vi "Updater Spartan INI.vi"(8 "error in (no error)":errorcluster, 10 "Spartan Server.ini":path, 11 "Copy Keys From INI":path) -> (0 "error out":errorcluster, 3 "Run as Service?":bool)   [LabVIEW 2011]
uses:
  Summitek EXT/OpenG EXT/file/file.llb/Valid Path - Traditional__ogtk.vi
  Summitek EXT/OpenG EXT/file/file.llb/File Exists - Scalar__ogtk.vi
  <vilib>/Utility/config.llb/Read Key (Boolean).vi
  <vilib>/Utility/config.llb/Read Key (String).vi
  <vilib>/Utility/config.llb/Write Key (String).vi
  <vilib>/Utility/config.llb/NI_LVConfig.lvlib
panel:
  # "This VI should run from TARGET root (e.g., \"<Program Files>\\Summitek\\Spartan\\\")\nwhenever the updater.exe runs.  It is used to put the \"Default Configuration.ini\"\ninto the \"Spartan Server.ini\" (while maintaining any previous relevant config values)."
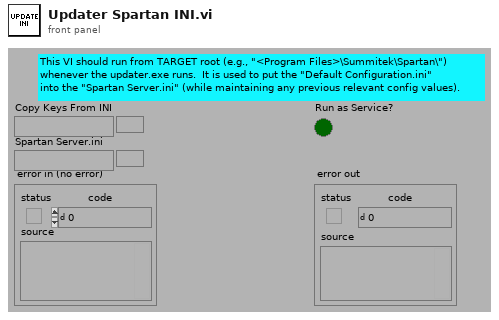
[diagram p1: front panel]
types:
  T1 = cluster{"Section":string, "Key":string, "Value":string}[]
  T2 = typedef "NI_LVConfig.lvlib/Config Data RefNum.ctl" = refnum<k1>
  T3 = cluster{"String":string, "String":string, "value":string}
  T4 = cluster{"String":string, "String":string, "value":string}[]
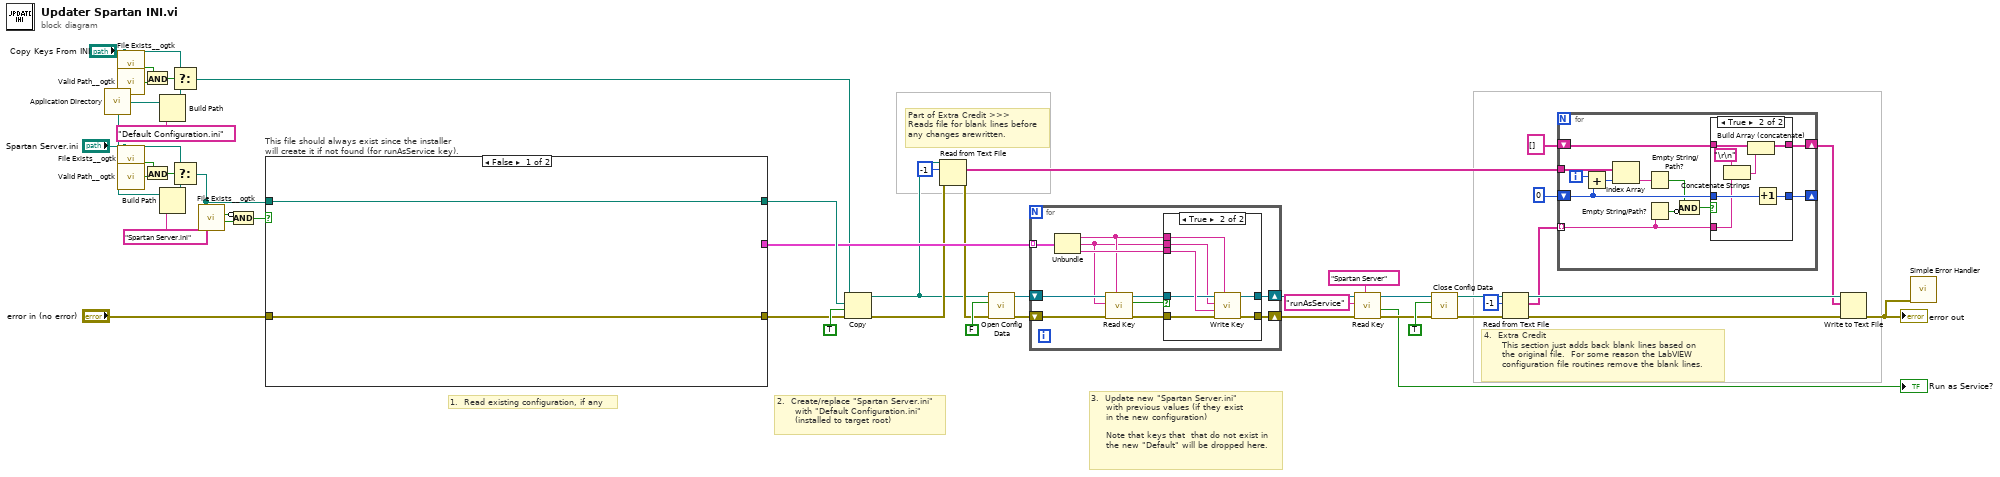
[diagram p0: block diagram]
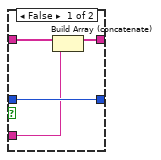
[diagram p2: hidden frame]
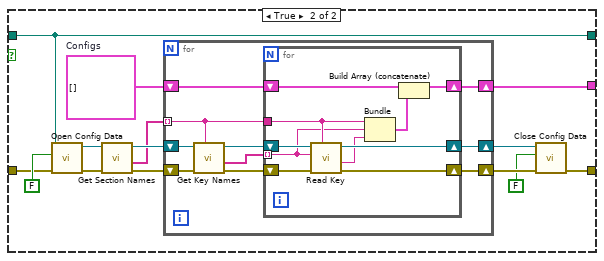
[diagram p4: hidden frame]
diagram:
  # "Part of Extra Credit >>>\nReads file for blank lines before\nany changes arewritten."
  # "4.  Extra Credit\n      This section just adds back blank lines based on\n      the original file.  For some reason the LabVIEW\n      configuration file routines remove the blank lines."
  # "3.  Update new \"Spartan Server.ini\"\n     with previous values (if they exist\n     in the new configuration)\n\n     Note that keys that  that do not exist in\n     the new \"Default\" will be dropped here."
  # "2.  Create/replace \"Spartan Server.ini\"\n      with \"Default Configuration.ini\"\n      (installed to target root)"
  # "1.  Read existing configuration, if any"
  n1 = call <vilib>:"Application Directory.vi"() -> ("Application Directory"=w14:path)
  n2 = call-poly "File Exists__ogtk.vi"("file path"="Copy Keys From INI") -> ("exists"=w7:bool)  [unwired: 6 in, 1 out]
  n3 = call-poly "Valid Path__ogtk.vi"("path"="Copy Keys From INI") -> ("valid"=w8:bool)
  n4 = call-poly "File Exists__ogtk.vi"("file path"="Spartan Server.ini") -> ("exists"=w5:bool)  [unwired: 6 in, 1 out]
  n5 = call-poly "Valid Path__ogtk.vi"("path"="Spartan Server.ini") -> ("valid"=w4:bool)
  n6 = And(x=w7, y=w8) -> (x .and. y?=w6:bool)
  n7 = And(x=w5, y=w4) -> (x .and. y?=w3:bool)
  n8 = Build Path(base path=w14, name or relative path="Default Configuration.ini") -> (appended path=w13:path)
  n9 = Build Path(base path=w14, name or relative path="Spartan Server.ini") -> (appended path=w11:path)
  n10 = Select(t="Copy Keys From INI", s=w6, f=w13) -> (s? t:f=w12:path)
  n11 = Select(t="Spartan Server.ini", s=w3, f=w11) -> (s? t:f=w10:path)
  n12 = call-poly "File Exists__ogtk.vi"("file path"=w10) -> ("is directory"=w47:bool, "exists"=w46:bool)  [unwired: 6 in]
  n13 = Compound Arithmetic op=AND(invert w47, w46) -> (w44:bool)
  n14 = case "This file should always exist since the installer will create it if not found (for runAsService key)." shown="False" w44 {
    tunnel: w10 -> [w49 w51]
    tunnel: "error in (no error)" -> [w50 w63]
    tunnel: [w50 w56] -> w41
    tunnel: [_ w52] -> w37
    tunnel: [w49 w51] -> w40
    frame False {
    }
    frame True {
      w53 = T1 []  # Configs
      n15 = call <vilib>:"Open Config Data.vi"("error in (no error)"=w63, "create file if necessary (T)"=FALSE, "configuration file path"=w51) -> ("error out"=w61:errorcluster, "refnum"=w62:T2)  [unwired: 6 in, 1 out]
      n16 = call <vilib>:"Get Section Names.vi"("error in (no error)"=w61, "refnum"=w62) -> ("error out"=w60:errorcluster, "section names"=w58:string[], "refnum out"=w59:T2)  [unwired: 7 in]
      n17 = for {
        shift-right: [w69] -> w57
        shift-left: w60 -> [w73]
        shift-right: [w70] -> w55
        shift-left: w59 -> [w74]
        tunnel: w58 -> [w68] mode=indexing
        shift-right: [w65] -> w52
        shift-left: w53 -> [w66]
        n18 = call <vilib>:"Get Key Names.vi"("section"=w68, "error in (no error)"=w73, "refnum"=w74) -> ("error out"=w71:errorcluster, "key names"=w67:string[], "refnum out"=w72:T2)  [unwired: 5 in, 1 out]
        n19 = for {
          shift-right: [w82] -> w69
          shift-left: w71 -> [w83]
          shift-right: [w81] -> w70
          shift-left: w72 -> [w84]
          tunnel: w68 -> [w80]
          tunnel: w67 -> [w79] mode=indexing
          shift-right: [w76] -> w65
          shift-left: w66 -> [w77]
          n20 = call-poly <vilib>:"Read Key.vi"("section"=w80, "error in (no error)"=w83, "key"=w79, "refnum"=w84) -> ("error out"=w82:errorcluster, "value"=w78:string, "refnum out"=w81:T2)  [unwired: 4 in, 1 out]
          n21 = Bundle("String"=w80, "String"=w79, "value"=w78) -> (w75:T3)  [unwired: 1 in]
          n22 = Build Array (concatenate)(w77, w75) -> (w76:T4)
        }
      }
      n23 = call <vilib>:"Close Config Data.vi"("error in (no error)"=w57, "write file if changed (T)"=FALSE, "refnum"=w55) -> ("error out"=w56:errorcluster)  [unwired: 7 in, 1 out]
    }
  }
  n24 = Copy(8:w41, 9:TRUE, 10:w40, 11:w12) -> (0:w34:errorcluster, 3:w32:path)  [unwired: 1 in, 1 out]
  n25 = Read from Text File(file (use dialog)=w32, count=-1, error in=w34) -> (text=w28:string[], error out=w33:errorcluster)  [unwired: 1 in, 2 out]
  n26 = call <vilib>:"Open Config Data.vi"("error in (no error)"=w33, "create file if necessary (T)"=FALSE, "configuration file path"=w32) -> ("error out"=w36:errorcluster, "refnum"=w35:T2)  [unwired: 6 in, 1 out]
  n27 = for {
    shift-right: [w94] -> w20
    shift-left: w36 -> [w91]
    shift-right: [w95] -> w21
    shift-left: w35 -> [w89]
    tunnel: w37 -> [w93] mode=indexing
    n28 = Unbundle(w93) -> ("Section"=w87:string, "Key"=w86:string, "Value"=w92:string)
    n29 = call-poly <vilib>:"Read Key.vi"("section"=w87, "error in (no error)"=w91, "key"=w86, "refnum"=w89) -> ("error out"=w90:errorcluster, "found?"=w85:bool, "refnum out"=w88:T2)  [unwired: 4 in, 1 out]
    n30 = case shown="True" w85 {
      tunnel: [w97 w104] -> w95
      tunnel: [w96 w103] -> w94
      tunnel: w92 -> [_ w102]
      tunnel: w90 -> [w96 w101]
      tunnel: w88 -> [w97 w100]
      tunnel: w87 -> [_ w99]
      tunnel: w86 -> [_ w98]
      frame False {
      }
      frame True {
        n31 = call-poly <vilib>:"Write Key.vi"("section"=w99, "error in (no error)"=w101, "value"=w102, "key"=w98, "refnum"=w100) -> ("error out"=w103:errorcluster, "refnum out"=w104:T2)  [unwired: 4 in, 1 out]
      }
    }
  }
  n32 = call-poly <vilib>:"Read Key.vi"("section"="Spartan Server", "error in (no error)"=w20, "key"="runAsService", "refnum"=w21) -> ("error out"=w18:errorcluster, "value"=→"Run as Service?":bool, "refnum out"=w19:T2)  [unwired: 4 in, 1 out]
  n33 = call <vilib>:"Close Config Data.vi"("error in (no error)"=w18, "write file if changed (T)"=TRUE, "refnum"=w19) -> ("error out"=w30:errorcluster, "file path"=w29:path)  [unwired: 7 in]
  n34 = Read from Text File(file (use dialog)=w29, count=-1, error in=w30) -> (text=w22:string[], error out=w26:errorcluster)  [unwired: 1 in, 2 out]
  n35 = for {
    tunnel: w28 -> [w113]
    shift-right: [w115] -> w23
    shift-left: string[] [] -> [w116]
    shift-right: [w114] -> _
    shift-left: 0 -> [w110]
    tunnel: w22 -> [w107] mode=indexing
    i -> [w111]
    n36 = Add(x=w111, y=w110) -> (x+y=w109:i32)
    n37 = Index Array(array=w113, index=w109) -> (element=w112:string)
    n38 = Empty String/Path?(string/path=w112) -> (empty?=w106:bool)
    n39 = Empty String/Path?(string/path=w107) -> (empty?=w108:bool)
    n40 = Compound Arithmetic op=AND(w106, invert w108) -> (w105:bool)
    n41 = case shown="True" w105 {
      tunnel: w116 -> [w120 w127]
      tunnel: [w119 w126] -> w115
      tunnel: w110 -> [w118 w125]
      tunnel: [w118 w124] -> w114
      tunnel: w107 -> [w117 w122]
      frame False {
        n42 = Build Array (concatenate)(w120, w117) -> (w119:string[])
      }
      frame True {
        n43 = Concatenate Strings("\r\n", w122) -> (w121:string)
        n44 = Build Array (concatenate)(w127, w121) -> (w126:string[])
        n45 = Increment(x=w125) -> (x+1=w124:i32)
      }
    }
  }
  n46 = Write to Text File(file (use dialog)=w29, text=w23, error in=w26) -> (error out=w9:errorcluster)  [unwired: 1 in, 2 out]
  "error out" <- w9
  n47 = call <vilib>:"Simple Error Handler.vi"("error in (no error)"=w9) -> ()  [unwired: 4 in, 5 out]
